vi "Log.vi"(11 "Data":T1) -> ()   [LabVIEW 2021]
panel:
  out "error out":errorcluster
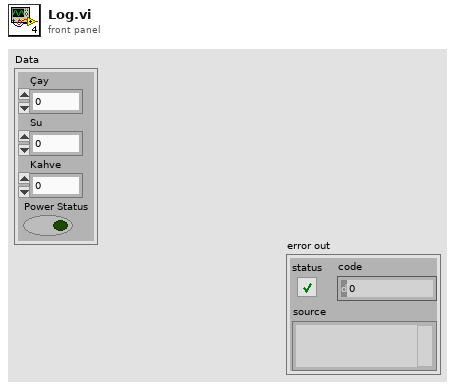
[diagram p1: front panel]
types:
  T1 = cluster{"Çay":dbl, "Su":dbl, "Kahve":dbl, "Power Status":bool}
  T2 = enum16{"open", "replace", "create", "open or create", "replace or create", "replace or create with confirmation"}
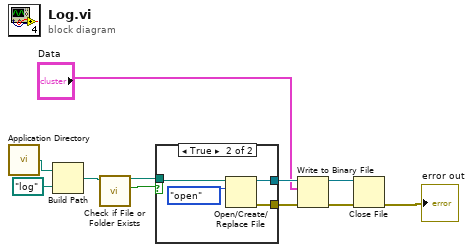
[diagram p0: block diagram]
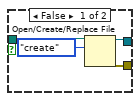
[diagram p2: hidden frame]
diagram:
  n1 = call <vilib>:"Application Directory.vi"() -> ("Application Directory"=w7:path)
  n2 = Build Path(base path=w7, name or relative path=path "log") -> (appended path=w5:path)
  n3 = call <vilib>:"Check if File or Folder Exists.vi"("path"=w5) -> ("file or folder exists?"=w4:bool, "dup path"=w3:path)  [unwired: 8 in, 1 out]
  n4 = case shown="True" w4 {
    tunnel: [w15 w19] -> w11
    tunnel: [w14 w18] -> w10
    tunnel: w3 -> [w13 w17]
    frame False {
      n5 = Open/Create/Replace File(file path (use dialog)=w13, operation (0:open)=T2."create") -> (refnum out=w15:refnum<file>, error out=w14:errorcluster)  [unwired: 4 in, 1 out]
    }
    frame True {
      n6 = Open/Create/Replace File(file path (use dialog)=w17, operation (0:open)=T2."open") -> (refnum out=w19:refnum<file>, error out=w18:errorcluster)  [unwired: 4 in, 1 out]
    }
  }
  n7 = Write to Binary File(file (use dialog)=w11, data="Data", error in=w10) -> (refnum out=w9:refnum<file>, error out=w8:errorcluster)  [unwired: 3 in, 1 out]
  n8 = Close File(refnum=w9, error in=w8) -> (error out=→"error out":errorcluster)  [unwired: 1 out]
